vi "Select Opp Kings Neighbours.vi"(9 "Opp King Cell Index":i32, 10 "Candidate Cells":i32[](array[numeric]), 11 "Parsed Board":T1) -> (2 "Moving to Opp. King's Neighbour?":bool, 3 "Selected Cell":i32)   [LabVIEW 2014]
uses:
  Typedefs/Parsed Board.ctl
  Dragon Tamers.lvlib
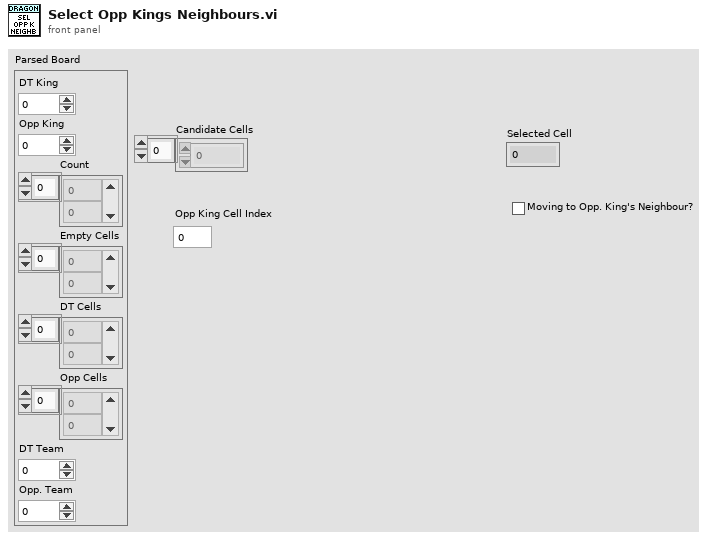
[diagram p1: front panel]
types:
  T1 = typedef "Dragon Tamers.lvlib/Parsed Board.ctl" = cluster{"DT King":i32, "Opp King":i32, "Count":i32[], "Empty Cells":i32[], "DT Cells":i32[], "Opp Cells":i32[], "DT Team":i32, "Opp. Team":i32}
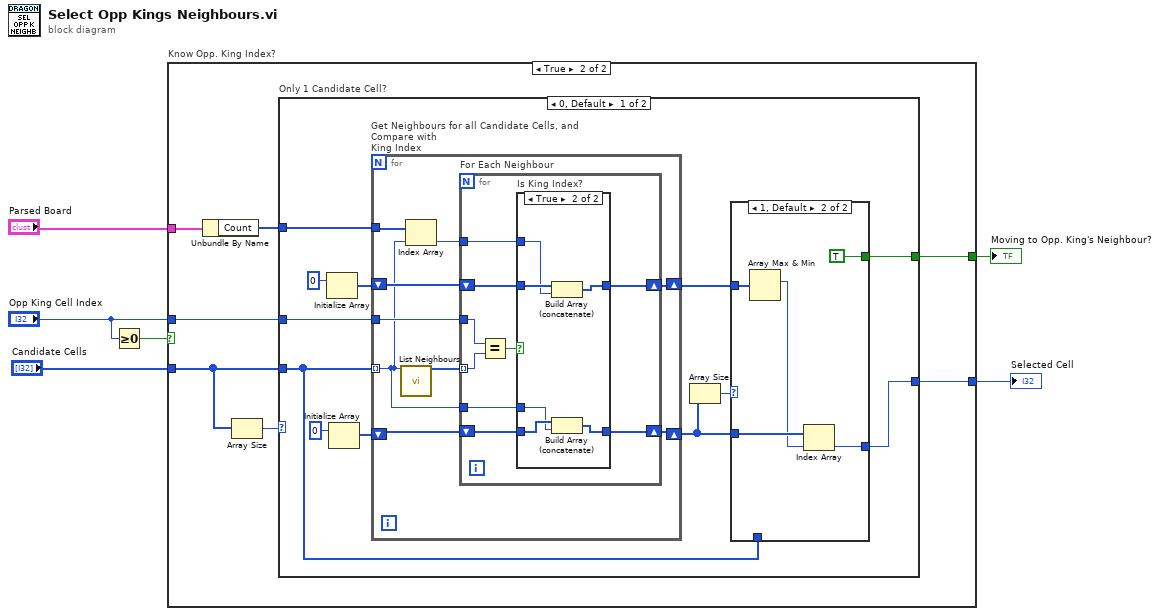
[diagram p0: block diagram]
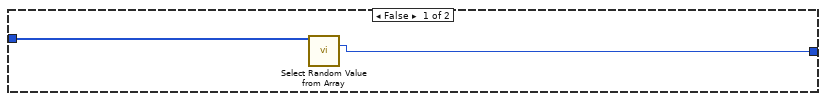
[diagram p2: hidden frame]
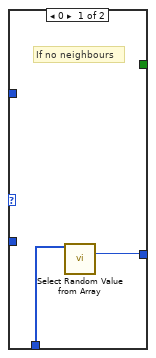
[diagram p3: hidden frame]
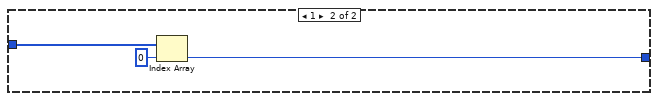
[diagram p5: hidden frame]
diagram:
  n1 = Greater Or Equal To 0?(x="Opp King Cell Index") -> (x >= 0?=w2:bool)
  n2 = case "Know Opp. King Index?" shown="True" w2 {
    tunnel: "Candidate Cells" -> [w8 w14]
    tunnel: "Opp King Cell Index" -> [_ w13]
    tunnel: [w7 w12] -> w5
    tunnel: "Parsed Board" -> [_ w11]
    tunnel: [_ w9] -> w1
    frame False {
      n3 = call "Select Random Value from Array.vi"("Array"=w8) -> ("Selected Value"=w7:i32)  [unwired: 11 in, 3 out]
    }
    frame True {
      n4 = Unbundle By Name(w11) -> ("Count"=w10:i32[])
      n5 = Array Size(array=w14) -> (size(s)=w15:i32)
      n6 = case "Only 1 Candidate Cell?" shown="0, Default" w15 {
        tunnel: w14 -> [w17 w63]
        tunnel: [w20 w61] -> w12
        tunnel: w13 -> [w27 _]
        tunnel: w10 -> [w22 _]
        tunnel: [w16 _] -> w9
        frame 0, Default {
          n7 = Initialize Array(0) -> (w23:i32[])  [unwired: 1 in]
          n8 = Initialize Array(0) -> (w25:i32[])  [unwired: 1 in]
          n9 = for "Get Neighbours for all Candidate Cells, and Compare with\nKing Index" {
            tunnel: w17 -> [w37] mode=indexing
            tunnel: w27 -> [w42]
            shift-right: [w40] -> w18
            shift-left: w25 -> [w41]
            shift-right: [w35] -> w21
            shift-left: w23 -> [w39]
            tunnel: w22 -> [w38]
            n10 = call "List Neighbours.vi"("Cell Index"=w37) -> ("Neighbours"=w43:i32[])  [unwired: 12 in, 2 out]
            n11 = Index Array(array=w38, index=w37) -> (element=w36:i32)
            n12 = for "For Each Neighbour" {
              tunnel: w43 -> [w49] mode=indexing
              tunnel: w42 -> [w52]
              shift-right: [w48] -> w40
              shift-left: w41 -> [w50]
              tunnel: w37 -> [w47]
              shift-right: [w44] -> w35
              shift-left: w39 -> [w46]
              tunnel: w36 -> [w45]
              n13 = Equal?(x=w52, y=w49) -> (x = y?=w51:bool)
              n14 = case "Is King Index?" shown="True" w51 {
                tunnel: w50 -> [w54 w60]
                tunnel: w47 -> [_ w59]
                tunnel: [w54 w58] -> w48
                tunnel: w46 -> [w53 w57]
                tunnel: w45 -> [_ w56]
                tunnel: [w53 w55] -> w44
                frame False {
                }
                frame True {
                  n15 = Build Array (concatenate)(w57, w56) -> (w55:i32[])
                  n16 = Build Array (concatenate)(w60, w59) -> (w58:i32[])
                }
              }
            }
          }
          n17 = Array Size(array=w18) -> (size(s)=w19:i32)
          n18 = case shown="1, Default" w19 {
            tunnel: w21 -> [_ w34]
            tunnel: w18 -> [_ w33]
            tunnel: [w28 w31] -> w20
            tunnel: w17 -> [w29 _]
            tunnel: [_ TRUE] -> w16
            frame 0 {
              # "If no neighbours"
              n19 = call "Select Random Value from Array.vi"("Array"=w29) -> ("Selected Value"=w28:i32)  [unwired: 11 in, 3 out]
            }
            frame 1, Default {
              n20 = Array Max & Min(array=w34) -> (max index (indices)=w32:i32)  [unwired: 3 out]
              n21 = Index Array(array=w33, index=w32) -> (element=w31:i32)
            }
          }
        }
        frame 1 {
          n22 = Index Array(array=w63, index=0) -> (element=w61:i32)
        }
      }
    }
  }
  "Selected Cell" <- w5
  "Moving to Opp. King's Neighbour?" <- w1
